vi "Generate Log Record.vi"(9 "data (null)":variant, 10 "message (\"\")":string, 11 "level (Internal)":T2=enum."Internal") -> (3 "log record":T1 {"timestamp" format="%<%x %.3X>T"})   [LabVIEW 2018, in "Logging.lvlib" / "Logger.lvclass"]
uses:
  Logger.lvclass
  Internal Log Levels.ctl
  Log Record.ctl
  Logging.lvlib
panel:
  # "Connector Pane"
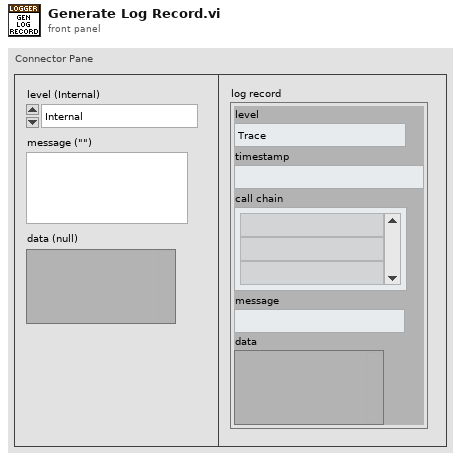
[diagram p1: front panel]
types:
  T1 = typedef "Logging.lvlib/Log Record.ctl" = cluster{"level":T2, "timestamp":timestamp, "call chain":string[], "message":string, "data":variant}
  T2 = typedef "Logging.lvlib/Internal Log Levels.ctl" = enum16{"Trace", "Debug", "Info", "Warning", "Error", "Critical", "Internal"}
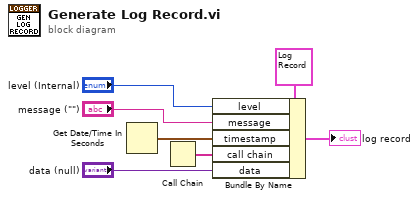
[diagram p0: block diagram]
diagram:
  n1 = Get Date/Time In Seconds() -> (seconds since 1Jan1904=w7:timestamp)
  n2 = Call Chain() -> (call chain=w6:string[])
  n3 = Bundle By Name(cluster=T1 {"level"=enum."Trace", "timestamp"=timestamp(0 s since 1904-01-01), "call chain"=[], "message"="", "data"=variant} ("output cluster 2"), "level"="level (Internal)", "message"="message (\"\")", "timestamp"=w7, "call chain"=w6, "data"="data (null)") -> (→"log record":T1)
